vi "dirRobot.vi"(4 "L2":dbl, 5 "L1":dbl, 6 "Angulo 2":dbl(knob), 7 "Angulo 1":dbl(knob)) -> (0 "y":dbl, 1 "x":dbl, 2 "y1":dbl, 3 "x1":dbl)   [LabVIEW 2014]
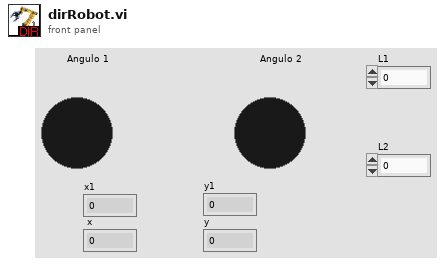
[diagram p1: front panel]
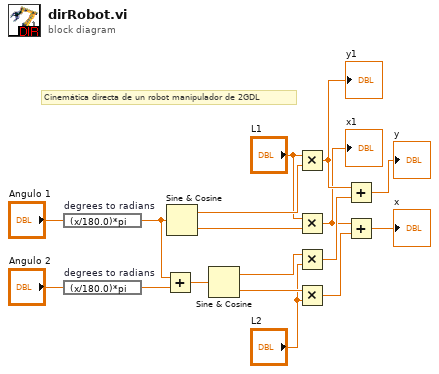
[diagram p0: block diagram]
diagram:
  # "Cinemática directa de un robot manipulador de 2GDL"
  n1 = expression code="(x/180.0)*pi" "degrees to radians"("Angulo 1") -> (w12:dbl)
  n2 = expression code="(x/180.0)*pi" "degrees to radians"("Angulo 2") -> (w11:dbl)
  n3 = Add(x=w12, y=w11) -> (x+y=w10:dbl)
  n4 = Sine & Cosine(0:w12) -> (1:w14:dbl, 2:w15:dbl)
  n5 = Sine & Cosine(0:w10) -> (1:w8:dbl, 2:w9:dbl)
  n6 = Multiply(x="L1", y=w14) -> (x*y=w5:dbl)
  "y1" <- w5
  n7 = Multiply(x="L1", y=w15) -> (x*y=w2:dbl)
  "x1" <- w2
  n8 = Multiply(x=w8, y="L2") -> (x*y=w6:dbl)
  n9 = Multiply(x=w9, y="L2") -> (x*y=w3:dbl)
  n10 = Add(x=w5, y=w6) -> (x+y=→"y":dbl)
  n11 = Add(x=w2, y=w3) -> (x+y=→"x":dbl)
